vi "DSF.Engine.Transfer Group.Offset Engine Pointers.vi"(8 "error in (no error)":errorcluster, 10 "engine base Pointer":refnum<class "DSF.Engine.Pointer.DBL.lvclass">, 11 "Transfer Group in":refnum<class "DSF.Engine.Transfer Group.lvclass">) -> (0 "error out":errorcluster, 3 "Transfer Group out":refnum<class "DSF.Engine.Transfer Group.lvclass">)   [LabVIEW 2017, in "DSF.Engine.lvlib" / "DSF.Engine.Transfer Group.lvclass"]
uses:
  DSF.Engine.Transfer Group.lvclass
  Pointer/DSF.Engine.Pointer.DBL.lvclass
  DSF.Engine.Transfer Group.lvclass/DSF.Engine.Transfer Group.ctl
  DSF.Engine.Transfer.lvclass
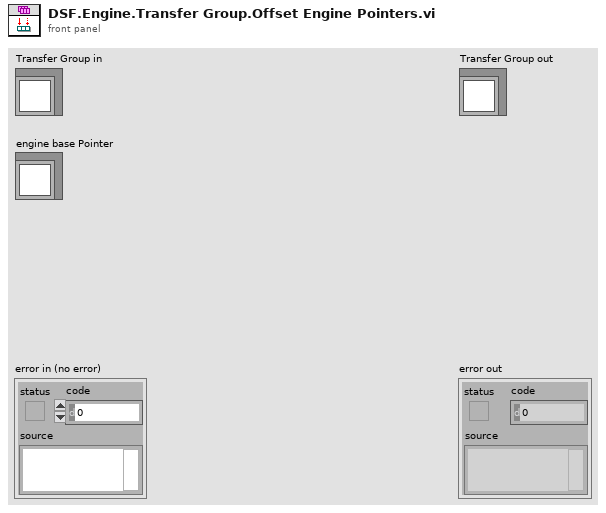
[diagram p1: front panel]
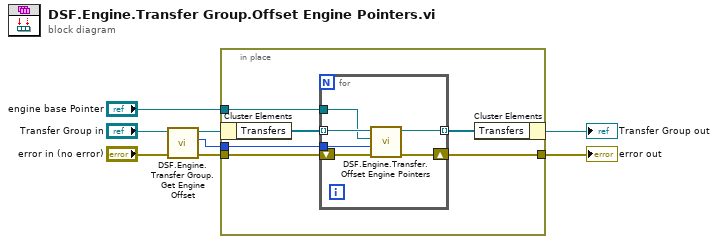
[diagram p0: block diagram]
diagram:
  n1 = call "DSF.Engine.Transfer Group.Get Engine Offset.vi"("Transfer Group in"="Transfer Group in") -> ("engine offset"=w1:u64, "Transfer Group out"=w2:refnum<class "DSF.Engine.Transfer Group.lvclass">)  [unwired: 9 in]
  n2 = in-place {
    in-place-border: [w11] -> w7
    in-place-border: "error in (no error)" -> [w10]
    in-place-border: "engine base Pointer" -> [w9]
    in-place-border: w1 -> [w8]
    n3 = in-place-cluster #1(w2) -> ("Transfers"=w13:refnum<class "DSF.Engine.Transfer.lvclass">[])
    n4 = for {
      tunnel: w13 -> [w19] mode=indexing
      tunnel: [w18] -> w12 mode=indexing
      shift-right: [w17] -> w11
      shift-left: w10 -> [w16]
      tunnel: w9 -> [w15]
      tunnel: w8 -> [w14]
      n5 = call "DSF.Engine.Transfer.Offset Engine Pointers.vi"("error in (no error)"=w16, "group engine offset"=w14, "engine base Pointer"=w15, "Transfer in"=w19) -> ("error out"=w17:errorcluster, "Transfer out"=w18:refnum<class "DSF.Engine.Transfer.lvclass">)  [unwired: 6 in]
    }
    n6 = in-place-cluster #1("Transfers"=w12) -> (→"Transfer Group out":refnum<class "DSF.Engine.Transfer Group.lvclass">)
  }
  "error out" <- w7
